vi "save.issue.vi"(8 "error in":errorcluster, 10 "issues path":path, 11 "issue data":T1) -> (0 "error out":errorcluster)   [LabVIEW 2024, in "manager_daemon.lvclass"]
uses:
  manager_daemon.lvclass
  manager_daemon.lvclass/manager_daemon.ctl
  CV_RESTful_Library/typedefs/cv_issue.generic_credit--cluster.ctl
  CV_RESTful_Library/CV_RESTful_Lib.lvlib
  CV_RESTful_Library/typedefs/cv_issue.associated_image--cluster.ctl
  CV_RESTful_Library/typedefs/cv_issue.person_credit--cluster.ctl
  CV_RESTful_Library/typedefs/local_issue--cluster.ctl
  <vilib>/addons/_JKI.lib/Serialization/JSON/JKI JSON Serialization.lvlib
  type_defs/IssueData--clustrer.ctl
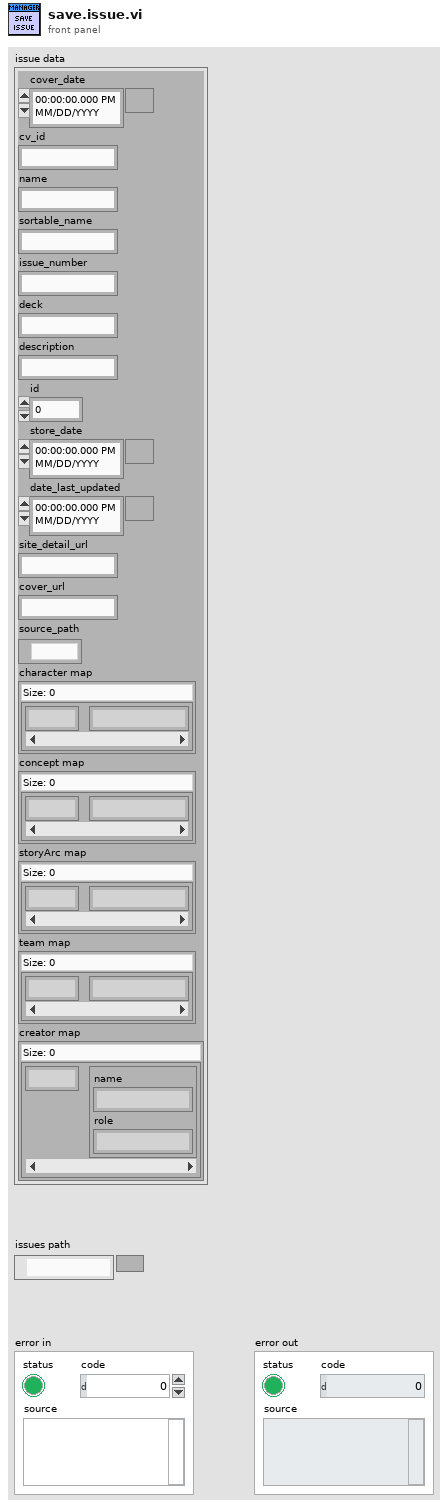
[diagram p1: front panel]
types:
  T1 = typedef "manager_daemon.lvclass/IssueData--clustrer.ctl" = cluster{"cover_date":timestamp, "cv_id":string, "name":string, "sortable_name":string, "issue_number":string, "deck":string, "description":string, "id":i32, "store_date":timestamp, "date_last_updated":timestamp, "site_detail_url":string, "cover_url":string, "source_path":path, "character map":map{i32, string}, "concept map":map{i32, string}, "storyArc map":map{i32, string}, "team map":map{i32, string}, "creator map":map{i32, cluster{"name":string, "role":string}}}
  T2 = typedef "CV_RESTful_Lib.lvlib/local_issue--cluster.ctl" = cluster{"cover_date":timestamp, "id":i32, "cv_id":string, "name":string, "sortable_name":string, "issue_number":string, "deck":string, "description":string, "volume":T3, "store_date":timestamp, "date_last_updated":timestamp, "site_detail_url":string, "cover_url":string, "associated_images":T4[], "characters":T3[], "concepts":T3[], "creators":T5[], "storyArcs":T3[], "teams":T3[]}
  T3 = typedef "CV_RESTful_Lib.lvlib/cv_issue.generic_credit--cluster.ctl" = cluster{"id":i32, "name":string}
  T4 = typedef "CV_RESTful_Lib.lvlib/cv_issue.associated_image--cluster.ctl" = cluster{"original_url":string, "id":i32}
  T5 = typedef "CV_RESTful_Lib.lvlib/cv_issue.person_credit--cluster.ctl" = cluster{"id":i32, "name":string, "role":string}
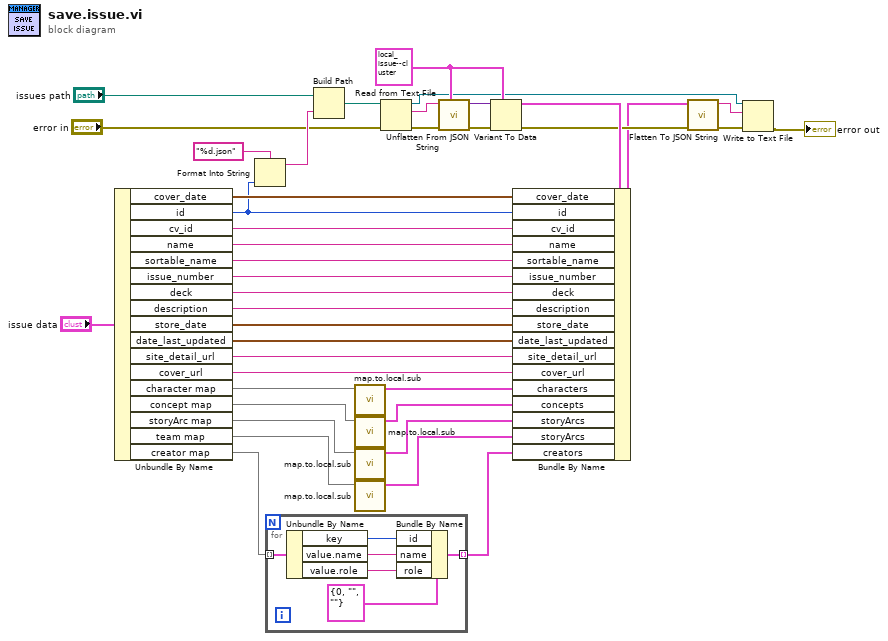
[diagram p0: block diagram]
diagram:
  w8 = T2 {"cover_date"=timestamp(0 s since 1904-01-01), "id"=0, "cv_id"="", "name"="", "sortable_name"="", "issue_number"="", "deck"="", "description"="", "volume"={"id"=0, "name"=""}, "store_date"=timestamp(0 s since 1904-01-01), "date_last_updated"=timestamp(0 s since 1904-01-01), "site_detail_url"="", "cover_url"="", "associated_images"=[], "characters"=[], "concepts"=[], "creators"=[], "storyArcs"=[], "teams"=[]} ("issue")
  n1 = Unbundle By Name("issue data") -> ("cover_date"=w39:timestamp, "id"=w17:i32, "cv_id"=w38:string, "name"=w37:string, "sortable_name"=w36:string, "issue_number"=w35:string, "deck"=w34:string, "description"=w33:string, "store_date"=w32:timestamp, "date_last_updated"=w31:timestamp, "site_detail_url"=w30:string, "cover_url"=w29:string, "character map"=w28:map{i32, string}, "concept map"=w26:map{i32, string}, "storyArc map"=w24:map{i32, string}, "team map"=w22:map{i32, string}, "creator map"=w20:map{i32, cluster{"name":string, "role":string}})
  n2 = Format Into String(format string="%d.json", w17) -> (resulting string=w15:string)  [unwired: 2 in, 1 out]
  n3 = for {
    tunnel: w20 -> [w46] mode=indexing
    tunnel: [w41] -> w19 mode=indexing
    n4 = Unbundle By Name(w46) -> ("key"=w44:i32, "value.name"=w43:string, "value.role"=w42:string)
    n5 = Bundle By Name(cluster=T5 {"id"=0, "name"="", "role"=""} ("character_credit"), "id"=w44, "name"=w43, "role"=w42) -> (w41:T5)
  }
  n6 = Build Path(base path="issues path", name or relative path=w15) -> (appended path=w14:path)
  n7 = call "map.to.local.sub.vi"("map in"=w28) -> ("array out"=w27:T3[])  [unwired: 10 in]
  n8 = call "map.to.local.sub.vi"("map in"=w26) -> ("array out"=w25:T3[])  [unwired: 10 in]
  n9 = call "map.to.local.sub.vi"("map in"=w24) -> ("array out"=w23:T3[])  [unwired: 10 in]
  n10 = call "map.to.local.sub.vi"("map in"=w22) -> ("array out"=w21:T3[])  [unwired: 10 in]
  n11 = Read from Text File(file (use dialog)=w14, error in="error in") -> (refnum out=w2:refnum<file>, text=w12:string, error out=w13:errorcluster)  [unwired: 2 in, 1 out]
  n12 = call <vilib>:"Unflatten From JSON String.vi"("Type and Defaults"=w8, "error in"=w13, "JSON String"=w12) -> ("error out"=w10:errorcluster, "Variant"=w9:variant)  [unwired: 7 in]
  n13 = Variant To Data(error in=w10, type=w8, Variant=w9) -> (data=w7:T2, error out=w6:errorcluster)
  n14 = Bundle By Name(cluster=w7, "cover_date"=w39, "id"=w17, "cv_id"=w38, "name"=w37, "sortable_name"=w36, "issue_number"=w35, "deck"=w34, "description"=w33, "store_date"=w32, "date_last_updated"=w31, "site_detail_url"=w30, "cover_url"=w29, "characters"=w27, "concepts"=w25, "storyArcs"=w23, "storyArcs"=w21, "creators"=w19) -> (w5:T2)
  n15 = call <vilib>:"Flatten To JSON String.vi"("error in"=w6, "Variant"=w5) -> ("error out"=w4:errorcluster, "JSON String"=w3:string)  [unwired: 8 in]
  n16 = Write to Text File(file (use dialog)=w2, text=w3, error in=w4) -> (error out=→"error out":errorcluster)  [unwired: 1 in, 2 out]
